vi "add single resource page.vi"(0 "Section Ptr in":T1 format="%.0x", 1 "cd resource name":string, 5 "channel type":T2, 7 "datatype":variant, 9 "name starts with...":string, 11 "error in (no error)":errorcluster) -> (4 "Section Ptr out":T1 format="%.0x", 15 "error out":errorcluster)   [LabVIEW 2016, in "FPGA RM System Definition API.lvlib"]
doc: "Adds a page to a Custom Device to reserve a single resource of the specified type."
uses:
  FPGA RM System Definition API.lvlib
  Channel Type.ctl
  <vilib>/NI Veristand/Custom Device API/Custom Device Item Ref.ctl
  <vilib>/NI VeriStand/Custom Device API/Custom Device API.lvlib
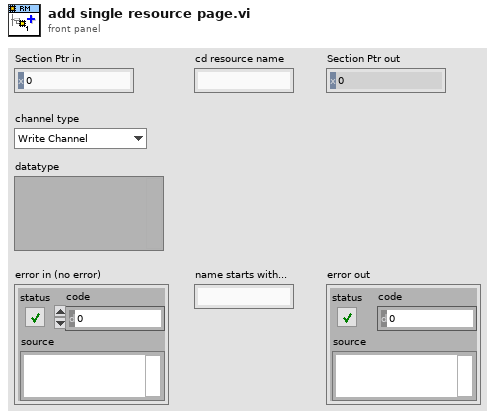
[diagram p1: front panel]
types:
  T1 = typedef "Custom Device API.lvlib/Custom Device Item Ref.ctl" = u64
  T2 = typedef "FPGA RM System Definition API.lvlib/Channel Type.ctl" = enum16{"Write Channel", "Read Channel", "Write Waveform", "Read Waveform"}
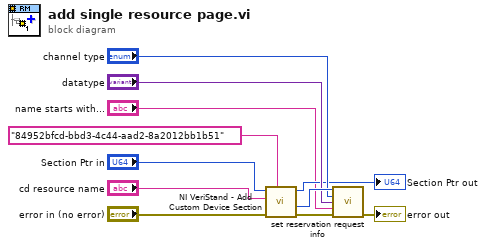
[diagram p0: block diagram]
diagram:
  n1 = call <vilib>:"NI VeriStand - Add Custom Device Section.vi"("GUID (Default Section)"="84952bfcd-bbd3-4c44-aad2-8a2012bb1b51", "error in (no error)"="error in (no error)", "Section Name"="cd resource name", "Parent Ref in"="Section Ptr in") -> ("error out"=w11:errorcluster, "Section Ptr"=w5:T1, "Parent Ref out"=→"Section Ptr out":T1)  [unwired: 4 in, 1 out]
  n2 = call "set reservation request info.vi"("Section Ptr"=w5, "channel type"="channel type", "datatype"="datatype", "Pattern"="name starts with...", "error in (no error)"=w11) -> ("error out"=→"error out":errorcluster)  [unwired: 9 in, 1 out]
